vi "generate id.vi"() -> (3 "id":string)   [LabVIEW 2016, in "client.lvlib" / "client.lvclass"]
uses:
  client.lvclass
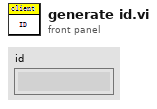
[diagram p1: front panel]
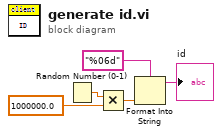
[diagram p0: block diagram]
diagram:
  n1 = Random Number (0-1)() -> (number: 0 to 1=w5:dbl)
  n2 = Multiply(x=w5, y=1000000.0) -> (x*y=w3:dbl)
  n3 = Format Into String(format string="%06d", w3) -> (resulting string=→"id":string)  [unwired: 2 in, 1 out]
